vi "示例 1.vi"() -> ()   [LabVIEW 2021]
panel:
  in  "N":i32
  out "Sum":i32
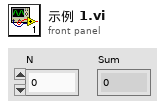
[diagram p1: front panel]
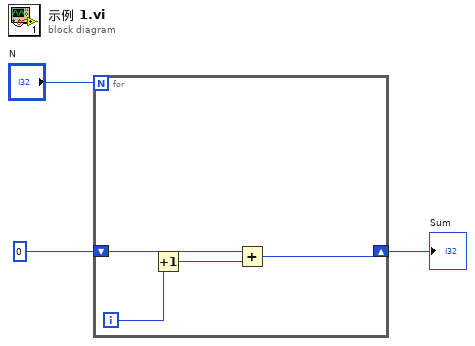
[diagram p0: block diagram]
diagram:
  n1 = for {
    N: "N" -> [_]
    shift-right: [w4] -> w1
    shift-left: 0 -> [w7]
    i -> [w6]
    n2 = Increment(x=w6) -> (x+1=w5:i32)
    n3 = Add(x=w7, y=w5) -> (x+y=w4:i32)
  }
  "Sum" <- w1
